vi "get_buffer.vi"(8 "error in (no error)":errorcluster, 9 "ulTimeoutInMs":u32, 11 "hCamera":u64) -> (0 "error out":errorcluster, 1 "output array":u16[][](array[numeric]), 2 "function return":i32, 3 "hCamera out":u64)   [LabVIEW 2013, in "Octoplus_LIDAR.lvlib"]
uses:
  <userlib>/Octoplus_LIDAR/Octoplus_LIDAR.lvlib
  <userlib>/Octoplus_LIDAR/CamCmosOctUsb3.dll
panel:
  out "size(s)":i32
  out "pixeltype":T1(ring)
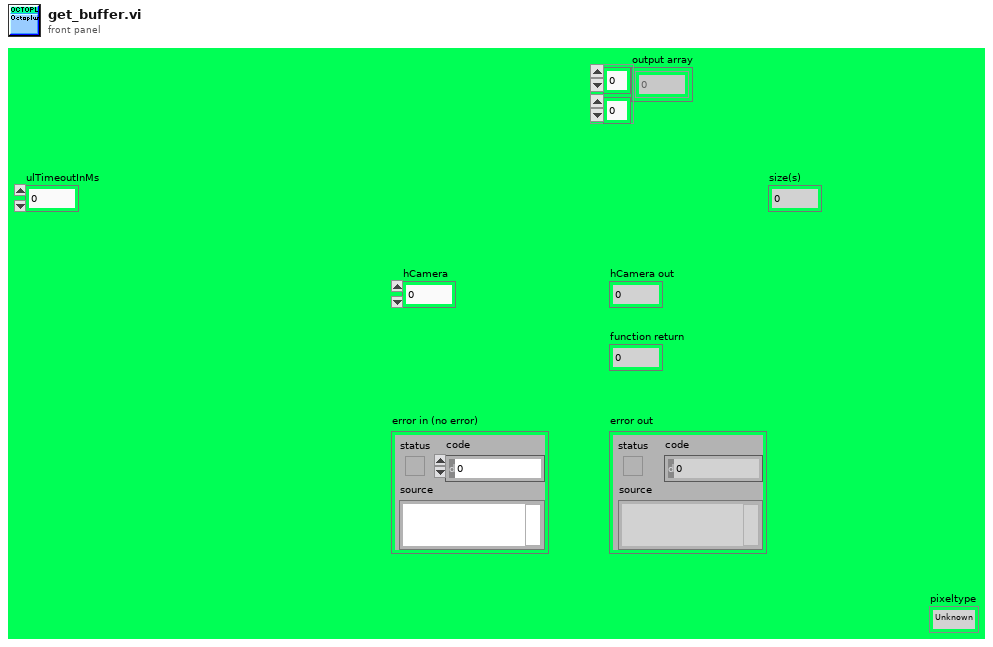
[diagram p1: front panel]
types:
  T1 = enum32{"Unknown", "Mono8", "Mono10", "Mono11", "Mono12"}
  T2 = cluster{"hBuffer":u64, "pData":u64, "ibufferSize":u64, "iImageSize":u64, "ioffsetX":u64, "iImageWidth":u64, "iImageHeight":u64, "eImagePixelType":u32, "filler1":u32, "iLinePitch":u64, "iiHorizontalFlip":u16, "filler2":u16, "filler3":u32, "iNbMissedTriggers":u64, "iNbLineLost":u64, "iNbImageAcquired":u64, "iFrameTriggerNbValidLines":u64}
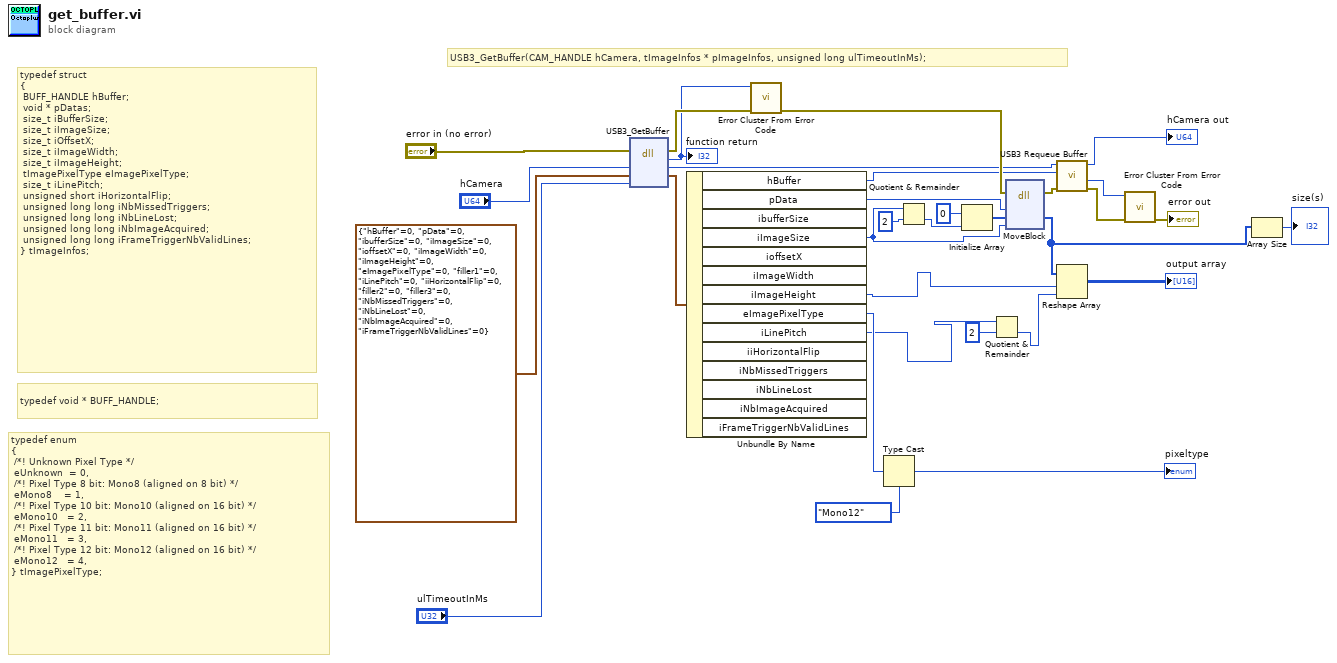
[diagram p0: block diagram]
diagram:
  # "typedef enum\n{\n\t/*! Unknown Pixel Type */\n\teUnknown  = 0,\n\t/*! Pixel Type 8 bit: Mono8 (aligned on 8 bit) */\n\teMono8    = 1,\n\t/*! Pixel Type 10 bit: Mono10 (aligned on 16 bit) */\n\teMono10   = 2,\n\t/*! Pixel Type 11 bit: Mono11 (aligned on 16 bit) */\n\teMono11   = 3,\n\t/*! Pixel Type 12 bit: Mono12 (aligned on 16 bit) */\n\teMono12   = 4,\n} tImagePixelType;"
  # "typedef void * BUFF_HANDLE;"
  # "typedef struct\n{\n\tBUFF_HANDLE\thBuffer;     \n\tvoid * pDatas; \n\tsize_t iBufferSize;\n\tsize_t iImageSize;\n\tsize_t iOffsetX;\n\tsize_t iImageWidth;\n\tsize_t iImageHeight;\n\ttImagePixelType eImagePixelType;\n\tsize_t iLinePitch;\n\tunsigned short iHorizontalFlip;\n\tunsigned long long iNbMissedTriggers;\n\tunsigned long long iNbLineLost;\n\tunsigned long long iNbImageAcquired;\n\tunsigned long long iFrameTriggerNbValidLines;\n} tImageInfos;"
  # "USB3_GetBuffer(CAM_HANDLE hCamera, tImageInfos * pImageInfos, unsigned long ulTimeoutInMs);"
  n1 = dll-call lib="C:/Program Files/National Instruments/LabVIEW 2013/user.lib/Octoplus_LIDAR/CamCmosOctUsb3.dll" fn="USB3_GetBuffer"(error in="error in (no error)", "hCamera"="hCamera", "pImageInfos"=T2 {"hBuffer"=0, "pData"=0, "ibufferSize"=0, "iImageSize"=0, "ioffsetX"=0, "iImageWidth"=0, "iImageHeight"=0, "eImagePixelType"=0, "filler1"=0, "iLinePitch"=0, "iiHorizontalFlip"=0, "filler2"=0, "filler3"=0, "iNbMissedTriggers"=0, "iNbLineLost"=0, "iNbImageAcquired"=0, "iFrameTriggerNbValidLines"=0} ("output cluster"), "ulTimeoutInMs"="ulTimeoutInMs") -> (error out=w22:errorcluster, "return type"=w21:i32, "hCamera"=w18:u64, "pImageInfos"=w28:T2)  [unwired: 3 in, 1 out]
  "function return" <- w21
  n2 = Unbundle By Name(w28) -> ("hBuffer"=w19:u64, "pData"=w23:u64, "iImageSize"=w6:u64, "iImageHeight"=w1:u64, "eImagePixelType"=w27:u32, "iLinePitch"=w5:u64)  [unwired: 8 out]
  n3 = call <vilib>:"Error Cluster From Error Code.vi"("error in (no error)"=w22, "error code (0)"=w21) -> ("error out"=w20:errorcluster)  [unwired: 7 in]
  n4 = Type Cast(type=T1."Mono12", x=w27) -> (*(type *) &x=→"pixeltype":T1)
  n5 = Quotient & Remainder(x=w6, y=u64 2) -> (floor(x/y)=w7:u64)  [unwired: 1 out]
  n6 = Initialize Array(u16 0, w7) -> (w24:u16[])
  n7 = Quotient & Remainder(x=w5, y=u64 2) -> (floor(x/y)=w2:u64)  [unwired: 1 out]
  n8 = dll-call lib="LabVIEW" fn="MoveBlock"(error in=w20, "Adress (Pointer)"=w23, "Destination"=w24, "Size"=w6) -> (error out=w17:errorcluster, "Destination"=w4:u16[])  [unwired: 5 in, 1 out]
  n9 = call <userlib>:"USB3 Requeue Buffer.vi"("error in (no error)"=w17, "hBuffer"=w19, "hCamera"=w18) -> ("error out"=w15:errorcluster, "function return"=w16:i32, "hCamera out"=→"hCamera out":u64)  [unwired: 5 in, 1 out]
  n10 = Reshape Array(w4, w1, w2) -> (→"output array":u16[][])
  n11 = call <vilib>:"Error Cluster From Error Code.vi"("error in (no error)"=w15, "error code (0)"=w16) -> ("error out"=→"error out":errorcluster)  [unwired: 7 in]
  n12 = Array Size(array=w4) -> (size(s)=→"size(s)":i32)
